vi "Close.vi"(8 "error in (no error)":errorcluster, 11 "ChannelService in":refnum<class "ChannelService.lvclass">) -> (0 "error out":errorcluster)   [LabVIEW 2020, in "Vecto.lvlib" / "ChannelService.lvclass"]
uses:
  ChannelService.lvclass
  ChannelService.lvclass/ChannelService.ctl
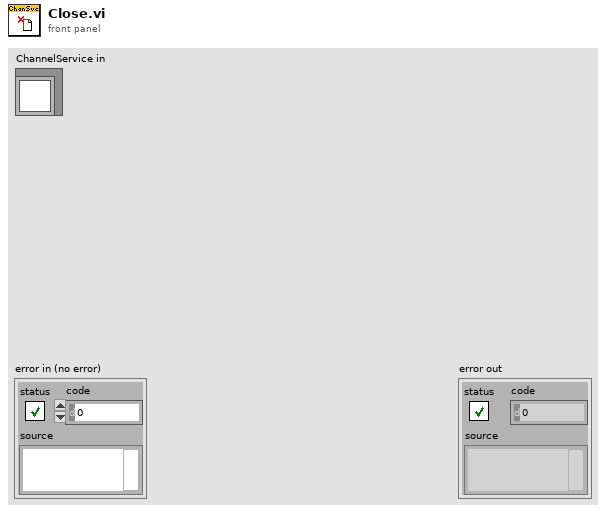
[diagram p1: front panel]
types:
  T1 = typedef "Vecto.lvlib/ChannelService.lvclass/Incoming Events.ctl" = cluster{"New Group":refnum<user-event>, "Close":refnum<user-event>}
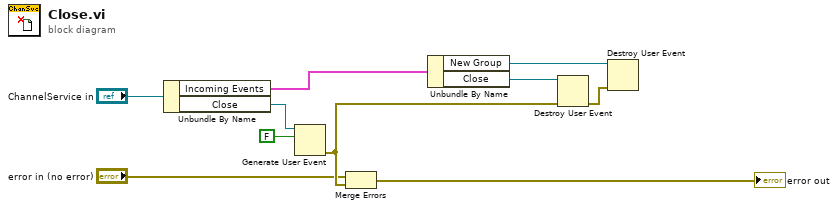
[diagram p0: block diagram]
diagram:
  n1 = Unbundle By Name("ChannelService in") -> ("Incoming Events"=w7:T1, "Close"=w9:refnum<user-event>)
  n2 = Generate User Event(user event=w9, event data cluster=FALSE ("event data")) -> (error out=w3:errorcluster)  [unwired: 2 in, 1 out]
  n3 = Merge Errors("error in (no error)", w3) -> (→"error out":errorcluster)
  n4 = Unbundle By Name(w7) -> ("New Group"=w5:refnum<user-event>, "Close"=w6:refnum<user-event>)
  n5 = Destroy User Event(user event=w6, error in=w3) -> (error out=w4:errorcluster)
  n6 = Destroy User Event(user event=w5, error in=w4) -> ()  [unwired: 1 out]
